vi "ziExample-Module-DAQ.vi"() -> ()   [LabVIEW 2009]
doc: "Control a Zurich instrument device via the LabOne Labview API. \nRequirements: Zurich Instruments MFLI, HF2 or UHFLI \nThis example shows how to start a DAQ trigger module and retrieve the Data.\n\n© Zurich Instruments AG, www.zhinst.com"
uses:
  <instrlib>/Zurich Instruments LabOne/Public/Modules/ziTypeModEnum.ctl
  <instrlib>/Zurich Instruments LabOne/Public/Modules/ziModSetValueDoubleArray.vi
  <instrlib>/Zurich Instruments LabOne/Public/Modules/ziModSetValueBinary.vi
  <instrlib>/Zurich Instruments LabOne/Public/Modules/ziModGetDoubleData.vi
  <instrlib>/Zurich Instruments LabOne/Public/Utility/ziTicksToS_vector.vi
  <instrlib>/Zurich Instruments LabOne/Zurich Instruments LabOne.lvlib
panel:
  in  "subscribe":string[](array[string])=["demods/0/sample.R", "demods/0/sample.Dio", "demods/0/sample.AuxIn1"] caption="Subscribe Paths"
  out "XY Graph":cluster{"Timestamp(s)":dbl[], "Value":dbl[]}[](graph)
  in  "stop":bool
  out "DoubleSample":T1
  in  "noofpoints":i32=10 caption="Number of Points"
  in  "duration":dbl=1.0 caption="Duration"
  out "Error Out":errorcluster
  in  "Address":string="DEV"
  out "Selected Device":string
  # "ziExample-Module-DAQ.vi\nRequirements: \n- HF2LI, UHFLI or MFLI \nsee block diagram for VI description"
  # "Tested Instruments:\n- HF2LI\n- UHFLI\n- MFLI"
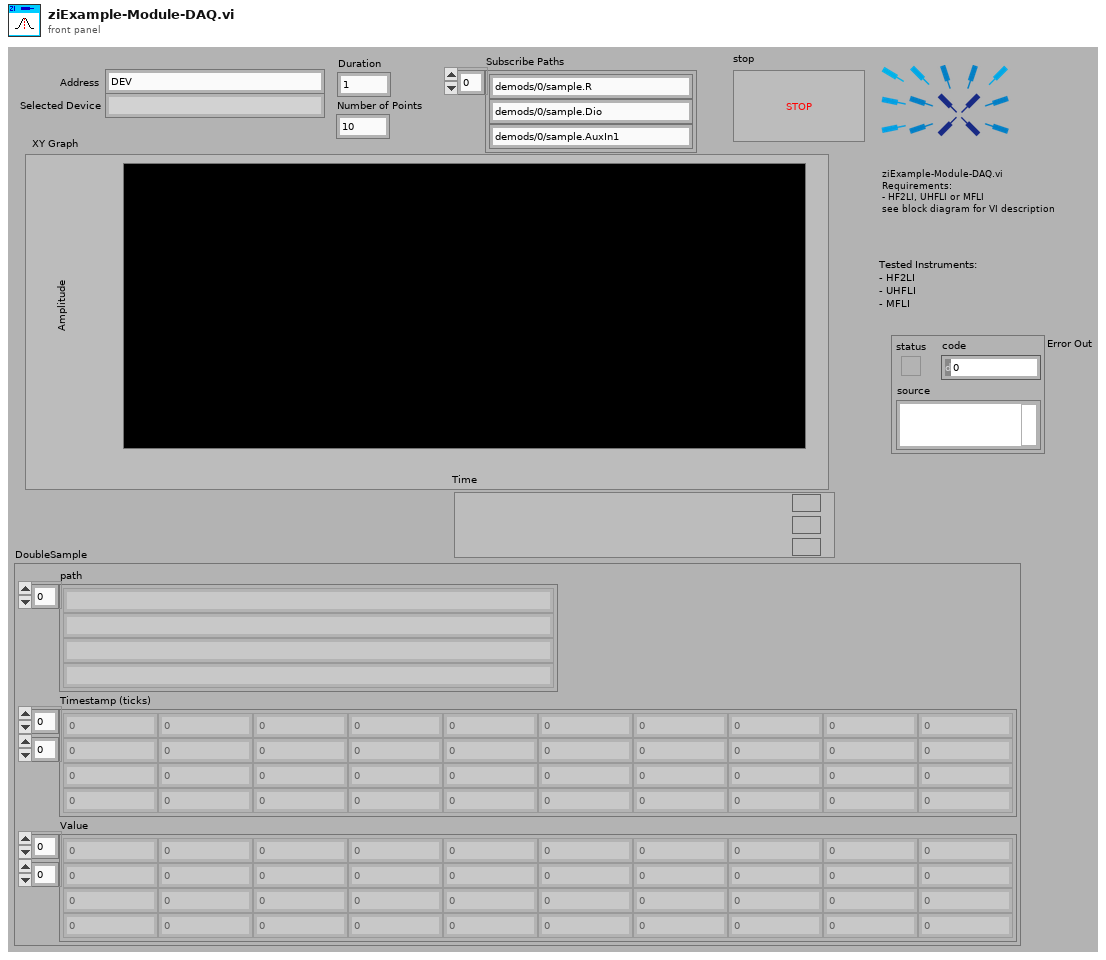
[diagram p1: front panel]
types:
  T1 = cluster{"path":string[], "Timestamp (ticks)":u64[][], "Value":dbl[][]}
  T2 = typedef "Zurich Instruments LabOne.lvlib/ziTypeModEnum.ctl" = u16
  T3 = typedef "Zurich Instruments LabOne.lvlib/ziTypeHandle.ctl" = cluster{"handleValid":bool, "Conn":u64, "Path Prefix":string, "Handle":u64, "Connected":bool, "Clockbase(s)":dbl}
  T4 = typedef "Zurich Instruments LabOne.lvlib/ziTypeModHandle.ctl" = cluster{"handleValid":bool, "Conn":u64, "ModHandle":u64, "moduleID":string, "Path Prefix":string}
  T5 = typedef "Zurich Instruments LabOne.lvlib/ziTypeModResults.ctl" = cluster{"PathArray":string[], "ValueType":T6, "NoOfResults":u64, "ziGenericHeader":T7[]}
  T6 = typedef "Zurich Instruments LabOne.lvlib/ziTypePollType.ctl" = enum16{"NONE", "DOUBLE_DATA", "INTEGER_DATA", "DEMOD_SAMPLE", "SCOPE_WAVE_HF2", "AUXIN_SAMPLE", "DIO_SAMPLE", "BYTE_ARRAY", "PWA_WAVE", "9", "10", "11", "12", "13", "14", "15", "TREE_CHANGE_DEPRI", "17", "ERROR", "19", "20", "21", "22", "23", "24", "25", "26", "27", "28", "29", "30", "31", "DOUBLE_DATA_TS", "INTEGER_DATA_TS", "34", "SCOPE_WAVE", "SCOPE_WAVE_EX", "37", "BYTE_ARRAY_TS", "39", "40", "41", "42", "43", "44", "45", "CNT_DATA", "47", "TREE_CHANGE", "49", "50", "51", "52", "53", "54", "55", "56", "57", "58", "59", "60", "61", "62", "63", "SWEEPER_DATA", "SPECTRUM_DATA", "ADVISOR_DATA", "VECTOR_DATA", "IMP_DATA"}
  T7 = typedef "Zurich Instruments LabOne.lvlib/ziTypeModGenericHeader.ctl" = cluster{"HeaderType":enum8{"HEADER_TYPE_NONE", "HEADER_TYPE_SWTRIGGER", "HEADER_TYPE_SWEEPER"}, "SampleFormat":u8, "SystemTime":timestamp, "CreatedTimeStamp":u64, "ChangedTimeStamp":u64, "Flags":u32, "ChunkSizeBytes":u64, "Name":string, "Status":u32, "GroupIndex":u32, "Color":u32, "ActiveRow":u32, "TriggerNumber":u64, "GridRows":u32, "GridCols":u32, "GridMode":u32, "GridOperation":u32, "GridDirection":u32, "GridRepetitions":u32, "GridColDelta":dbl, "GridColOffset":dbl, "GridRowDelta":dbl, "GridRowOffset":dbl, "Bandwidth":dbl, "Center":dbl, "Nenbw":dbl}
  T8 = typedef "Zurich Instruments LabOne.lvlib/ziTypeDoubleDataTS.ctl" = cluster{"Timestamp (ticks)":u64[], "Value":dbl[]}
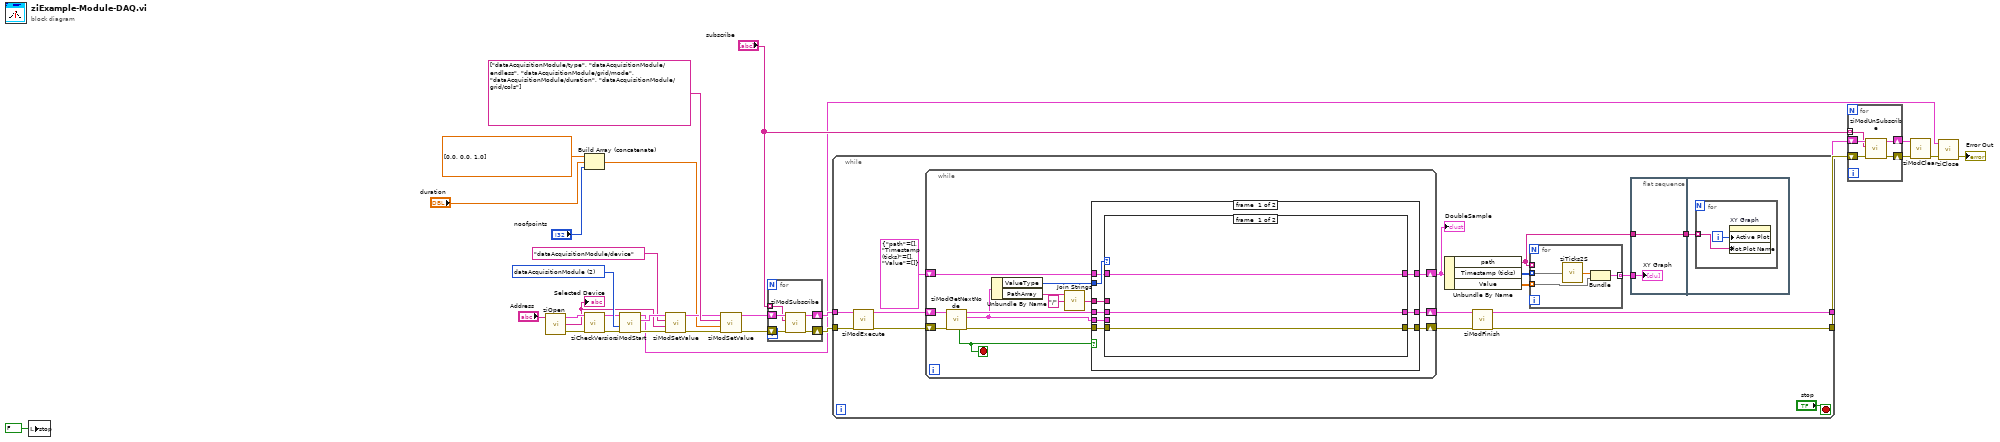
[diagram p0: block diagram]
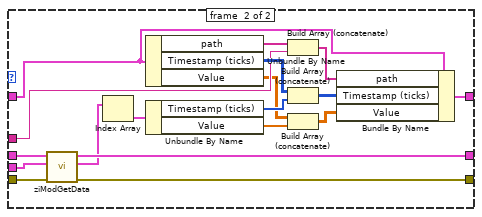
[diagram p2: hidden frame]
diagram:
  w9 = T2 2 items=["sweep", "scopeModule", "dataAcquisitionModule", "pidAdvisor", "awgModule", "impedanceModule", "multiDeviceSyncModule", "zoomFFT", "trigger", "deviceSettings", "record"] ("module Id")
  n1 = local write "stop"(FALSE ("run")) -> ()
  n2 = call <instrlib>:"ziOpen.vi"("Address"="Address") -> ("Error Out"=w23:errorcluster, "Selected Device"=w6:string, "HandleOut"=w24:T3)  [unwired: 1 in, 2 out]
  "Selected Device" <- w6
  n3 = Build Array (concatenate)(dbl[] [0.0, 0.0, 1.0], "duration", "noofpoints") -> (w10:dbl[])
  n4 = call <instrlib>:"ziCheckVersion.vi"("Handle In"=w24, "Error In"=w23) -> ("Handle Out"=w8:T3, "Error Out"=w7:errorcluster)  [unwired: 11 in, 1 out]
  n5 = call <instrlib>:"ziModStart.vi"("Error In"=w7, "module Id"=w9, "Handle In"=w8) -> ("Error Out"=w25:errorcluster, "ModHandle Out"=w26:T4, "Handle Out"=w1:T3)  [unwired: 6 in]
  n6 = call-poly <instrlib>:"ziModSetValue.vi"("Error In"=w25, "Data"=w6, "Path"="dataAcquisitionModule/device", "ModHandle In"=w26) -> ("Error Out"=w18:errorcluster, "ModHandle Out"=w19:T4)  [unwired: 6 in]
  n7 = call-poly <instrlib>:"ziModSetValue.vi"("Error In"=w18, "Values"=w10, "Paths"=string[] ["dataAcquisitionModule/type", "dataAcquisitionModule/endless", "dataAcquisitionModule/grid/mode", "dataAcquisitionModule/duration", "dataAcquisitionModule/grid/cols"], "ModHandle In"=w19) -> ("Error Out"=w14:errorcluster, "ModHandle Out"=w15:T4)  [unwired: 6 in]
  n8 = for {
    tunnel: "subscribe" -> [w31] mode=indexing
    shift-right: [w35] -> w17
    shift-left: w15 -> [w33]
    shift-right: [w34] -> w16
    shift-left: w14 -> [w32]
    n9 = call <instrlib>:"ziModSubscribe.vi"("Error In"=w32, "Path"=w31, "ModHandle In"=w33) -> ("Error Out"=w34:errorcluster, "ModHandle Out"=w35:T4)  [unwired: 6 in]
  }
  n10 = while {
    tunnel: [w38] -> w22
    tunnel: [w49] -> w21
    tunnel: w17 -> [w48]
    tunnel: w16 -> [w47]
    stop <- "stop" stop-if-true
    n11 = call <instrlib>:"ziModExecute.vi"("Error In"=w47, "ziModHandle In"=w48) -> ("Error Out"=w45:errorcluster, "ziModHandle Out"=w46:T4)  [unwired: 6 in, 1 out]
    n12 = while {
      shift-right: [w69] -> w50
      shift-left: w46 -> [w73]
      shift-right: [w70] -> w51
      shift-left: w45 -> [w74]
      shift-right: [w62] -> w42
      shift-left: T1 {"path"=[], "Timestamp (ticks)"=[], "Value"=[]} ("DoubleSample") -> [w63]
      stop <- w68 stop-if-true
      n13 = call <instrlib>:"ziModGetNextNode.vi"("Error In"=w74, "ModHandle In"=w73) -> ("Error Out"=w71:errorcluster, "ModResults"=w67:T5, "ModHandle Out"=w72:T4, "NoData"=w68:bool)  [unwired: 6 in]
      n14 = Unbundle By Name(w67) -> ("ValueType"=w64:T6, "PathArray"=w61:string[])
      n15 = call <vilib>:"Join Strings.vi"("Separator (,)"="/", "Strings In"=w61) -> ("String"=w65:string)  [unwired: 1 in]
      n16 = case shown="False" w68 {
        tunnel: w67 -> [w83 _]
        tunnel: w72 -> [w82 w107]
        tunnel: w71 -> [w81 w106]
        tunnel: [w80 w106] -> w70
        tunnel: [w79 w107] -> w69
        tunnel: w65 -> [w75 _]
        tunnel: w64 -> [w78 _]
        tunnel: w63 -> [w77 w105]
        tunnel: [w76 w105] -> w62
        frame #0 {
          n17 = case shown="\"DOUBLE_DATA_TS\"" w78 {
            tunnel: w82 -> [w86 w101]
            tunnel: w83 -> [_ w100]
            tunnel: w81 -> [w85 w102]
            tunnel: [w85 w103] -> w80
            tunnel: [w86 w104] -> w79
            tunnel: w77 -> [w84 w90]
            tunnel: [w84 w91] -> w76
            tunnel: w75 -> [_ w93]
            frame #0 {
            }
            frame #1 {
              n18 = call-poly <instrlib>:"ziModGetData.vi"("Error In"=w102, "ModResults"=w100, "ModHandle In"=w101) -> ("Error Out"=w103:errorcluster, "DoubleSample"=w99:T8[], "ModHandle Out"=w104:T4)  [unwired: 4 in, 2 out]
              n19 = Index Array(array=w99) -> (element=w98:T8)  [unwired: 1 in]
              n20 = Unbundle By Name(w90) -> ("path"=w94:string[], "Timestamp (ticks)"=w97:u64[][], "Value"=w89:dbl[][])
              n21 = Unbundle By Name(w98) -> ("Timestamp (ticks)"=w96:u64[], "Value"=w88:dbl[])
              n22 = Build Array (concatenate)(w94, w93) -> (w92:string[])
              n23 = Build Array (concatenate)(w97, w96) -> (w95:u64[][])
              n24 = Build Array (concatenate)(w89, w88) -> (w87:dbl[][])
              n25 = Bundle By Name(cluster=w90, "path"=w92, "Timestamp (ticks)"=w95, "Value"=w87) -> (w91:T1)
            }
          }
        }
        frame #1 {
        }
      }
    }
    "DoubleSample" <- w42
    n26 = Unbundle By Name(w42) -> ("path"=w36:string[], "Timestamp (ticks)"=w41:u64[][], "Value"=w40:dbl[][])
    n27 = call <instrlib>:"ziModFinish.vi"("Error In"=w51, "ziModHandle In"=w50) -> ("Error Out"=w38:errorcluster, "ziModHandle Out"=w49:T4)  [unwired: 7 in]
    n28 = for {
      tunnel: w41 -> [w58] mode=indexing
      tunnel: w40 -> [w60] mode=indexing
      tunnel: [w59] -> w39 mode=indexing
      tunnel: w36 -> [_] mode=indexing
      n29 = call-poly <instrlib>:"ziTicks2S.vi"("Timestamp (ticks)"=w58) -> ("Timestamp(s)"=w57:dbl[])  [unwired: 2 in, 2 out]
      n30 = Bundle("Timestamp(s)"=w57, "Value"=w60) -> (w59:cluster{"Timestamp(s)":dbl[], "Value":dbl[]})  [unwired: 1 in]
    }
    n31 = flat-sequence {
      tunnel: w39 -> [w53]
      tunnel: [w52] -> w37
      tunnel: w36 -> [w52]
      tunnel: w37 -> [w54]
      frame #0 {
        "XY Graph" <- w53
      }
      frame #1 {
        n32 = for {
          tunnel: w54 -> [w56] mode=indexing
          i -> [w55]
          n33 = property on="XY Graph" class="XYGraph (strict)"("Active Plot"=w55, "Plot.Plot Name"=w56) -> ()  [unwired: 2 in, 2 out]
        }
      }
    }
  }
  n34 = for {
    tunnel: "subscribe" -> [w108] mode=indexing
    shift-right: [w111] -> w28
    shift-left: w21 -> [w109]
    shift-right: [w112] -> w29
    shift-left: w22 -> [w110]
    n35 = call <instrlib>:"ziModUnSubscribe.vi"("Error In"=w110, "Path (\"/\")"=w108, "ModHandle In"=w109) -> ("Error Out"=w112:errorcluster, "ModHandle Out"=w111:T4)  [unwired: 7 in]
  }
  n36 = call <instrlib>:"ziModClear.vi"("Error In"=w29, "ziModHandle In"=w28) -> ("Error Out"=w4:errorcluster)  [unwired: 7 in, 1 out]
  n37 = call <instrlib>:"ziClose.vi"("Error In"=w4, "Handle In"=w1) -> ("Error Out"=→"Error Out":errorcluster)  [unwired: 2 in, 1 out]
